vi "Status updated--constant.vi"() -> (3 "Topic":string[](array[string]))   [LabVIEW 2016, in "MQTT_Client.lvlib"]
uses:
  MQTT_Client.lvlib
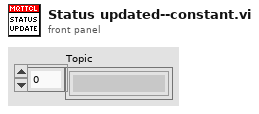
[diagram p1: front panel]
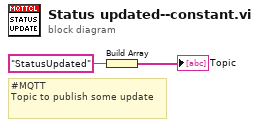
[diagram p0: block diagram]
diagram:
  # "#MQTT   \nTopic to publish some update"
  n1 = Build Array("StatusUpdated" ("Topic")) -> (→"Topic":string[])
